vi "Auto_Contorl.vi"() -> (0 "Auto_Contorl":cluster{"Auto_Selection":T1, "Auto_Enable":bool})   [LabVIEW 2015]
uses:
  Auto/Auto_Selection.ctl
  Auto/Auto_Global.vi
panel:
  out "Waveform Chart":i16(graph)
  in  "Manual_Auto_Enable":bool
  in  "Auto_Selection":T1
  in  "Manual_Auto":bool
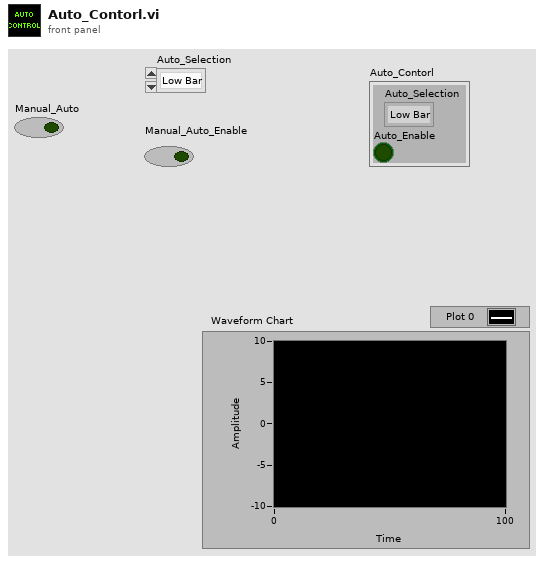
[diagram p1: front panel]
types:
  T1 = typedef "Auto_Selection.ctl" = enum16{"Low Bar", "Rough Terrain", "Rock Wall", "Ramparts", "Moat", "Cheval de Frise", "Portcullis", "None", "One  Ball"}
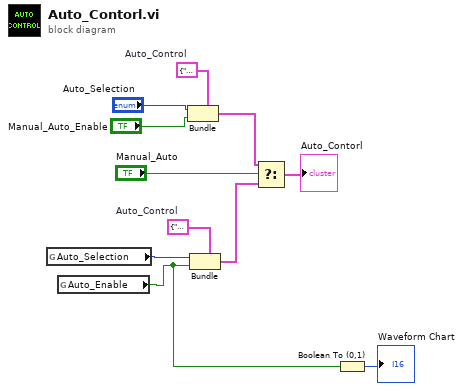
[diagram p0: block diagram]
diagram:
  w4 = cluster{"Auto_Selection":T1, "Auto_Enable":bool} {"Auto_Selection"=enum."Low Bar", "Auto_Enable"=FALSE}  # Auto_Control
  w5 = cluster{"Auto_Selection":T1, "Auto_Enable":bool} {"Auto_Selection"=enum."Low Bar", "Auto_Enable"=FALSE}  # Auto_Control
  n1 = global read "Auto_Global.vi" "Auto_Selection"() -> (w9:T1)
  n2 = global read "Auto_Global.vi" "Auto_Enable"() -> (w1:bool)
  n3 = Bundle(cluster=w5, "Auto_Selection"="Auto_Selection", "Auto_Enable"="Manual_Auto_Enable") -> (w6:cluster{"Auto_Selection":T1, "Auto_Enable":bool})
  n4 = Bundle(cluster=w4, "Auto_Selection"=w9, "Auto_Enable"=w1) -> (w10:cluster{"Auto_Selection":T1, "Auto_Enable":bool})
  n5 = Select(t=w6, s="Manual_Auto", f=w10) -> (s? t:f=→"Auto_Contorl":cluster{"Auto_Selection":T1, "Auto_Enable":bool})
  n6 = Boolean To (0,1)(Boolean=w1) -> (0, 1=→"Waveform Chart":i16)
